vi "dfd_Classical Order Estimation Param Validation.vi"(6 "fs [Hz]":dbl=1.0 format="%.2f", 7 "filter type":T3(ring), 8 "error in (no error)":errorcluster, 10 "ripple specs":T1={"passband"=0.0, "stopband"=0.0, "dB/linear? (T: dB)"=TRUE}, 11 "freq specs [Hz]":T2) -> (0 "error out":errorcluster, 2 "dup ripple specs":T1={"passband"=0.0, "stopband"=0.0, "dB/linear? (T: dB)"=TRUE}, 3 "dup freq specs [Hz]":T2)   [LabVIEW 2017, in "NI_DigFilterLicensed.lvlib"]
doc: "Validates the parameters for order estimation."
uses:
  <vilib>/addons/Digital Filter Design/NI_DigFilterLicensed.lvlib
  <vilib>/addons/Digital Filter Design/_Objects.llb/DFD Filter Frequence Specification (Design).ctl
  <vilib>/addons/Digital Filter Design/_Objects.llb/DFD Filter Ripple Specification (Design).ctl
  <vilib>/addons/Digital Filter Design/_Misc.llb/dfd_Error Handlers (Multiple).vi
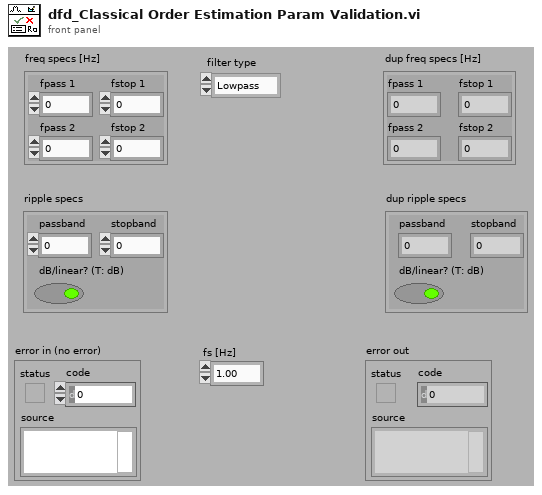
[diagram p1: front panel]
types:
  T1 = typedef "NI_DigFilterLicensed.lvlib/DFD Filter Ripple Specification (Design).ctl" = cluster{"passband":dbl, "stopband":dbl, "dB/linear? (T: dB)":bool}
  T2 = typedef "NI_DigFilterLicensed.lvlib/DFD Filter Frequence Specification (Design).ctl" = cluster{"fpass 1":dbl, "fstop 1":dbl, "fpass 2 ":dbl, "fstop 2":dbl}
  T3 = enum16{"Lowpass", "Highpass", "Bandpass", "Bandstop"}
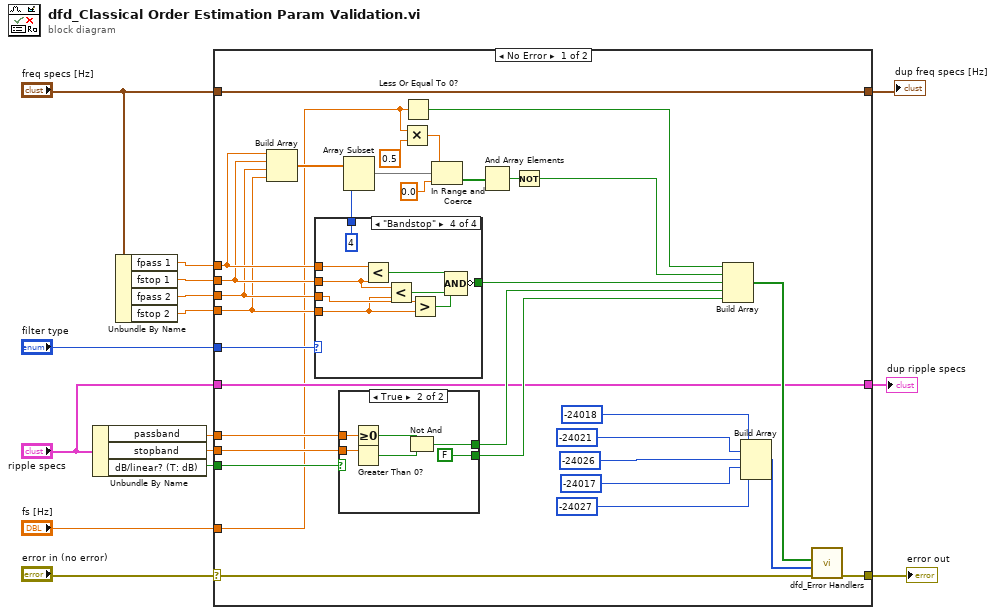
[diagram p0: block diagram]
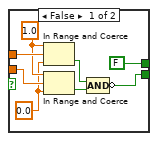
[diagram p2: hidden frame]
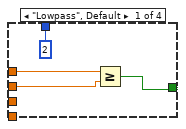
[diagram p3: hidden frame]
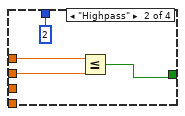
[diagram p4: hidden frame]
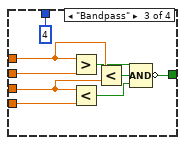
[diagram p5: hidden frame]
diagram:
  n1 = Unbundle By Name("ripple specs") -> ("passband"=w8:dbl, "stopband"=w7:dbl, "dB/linear? (T: dB)"=w9:bool)
  n2 = Unbundle By Name("freq specs [Hz]") -> ("fpass 1"=w13:dbl, "fstop 1"=w12:dbl, "fpass 2"=w11:dbl, "fstop 2"=w10:dbl)
  n3 = case shown="No Error" "error in (no error)" {
    selector: "error in (no error)" -> [w32 w89]
    tunnel: "fs [Hz]" -> [w26 _]
    tunnel: "filter type" -> [w48 _]
    tunnel: w13 -> [w42 _]
    tunnel: w12 -> [w41 _]
    tunnel: w11 -> [w40 _]
    tunnel: w10 -> [w39 _]
    tunnel: w9 -> [w45 _]
    tunnel: w8 -> [w44 _]
    tunnel: w7 -> [w43 _]
    tunnel: [w31 w89] -> w6
    tunnel: [w30 _] -> w3
    tunnel: "freq specs [Hz]" -> [w30 _]
    tunnel: "ripple specs" -> [w29 _]
    tunnel: [w29 _] -> w1
    frame No Error {
      n4 = Build Array(w42, w41, w40, w39) -> (w28:dbl[])
      n5 = case shown="\"Bandstop\"" w48 {
        tunnel: w42 -> [w66 w70 w77 w88]
        tunnel: w41 -> [w65 w69 w79 w87]
        tunnel: w40 -> [_ _ w76 w86]
        tunnel: w39 -> [_ _ w78 w80]
        tunnel: [w64 w68 w72 w82] -> w47
        tunnel: [2 2 4 4] -> w27
        frame "Lowpass", Default {
          n6 = Greater Or Equal?(x=w66, y=w65) -> (x >= y?=w64:bool)
        }
        frame "Highpass" {
          n7 = Less Or Equal?(x=w70, y=w69) -> (x <= y?=w68:bool)
        }
        frame "Bandpass" {
          n8 = Greater?(x=w77, y=w79) -> (0:w75:bool)
          n9 = Less?(x=w76, y=w78) -> (x < y?=w73:bool)
          n10 = Less?(x=w77, y=w76) -> (x < y?=w74:bool)
          n11 = Compound Arithmetic op=AND(w75, w74, w73) -> (invert w72:bool)
        }
        frame "Bandstop" {
          n12 = Less?(x=w88, y=w87) -> (x < y?=w85:bool)
          n13 = Less?(x=w87, y=w80) -> (x < y?=w84:bool)
          n14 = Greater?(x=w86, y=w80) -> (0:w83:bool)
          n15 = Compound Arithmetic op=AND(w85, w84, w83) -> (invert w82:bool)
        }
      }
      n16 = case shown="True" w45 {
        tunnel: w44 -> [w54 w62]
        tunnel: w43 -> [w55 w61]
        tunnel: [FALSE w58] -> w36
        tunnel: [w49 FALSE] -> w35
        frame False {
          w52 = 0.0 ("lower limit")
          w53 = 1.0 ("y")
          n17 = In Range and Coerce(upper limit=w53, x=w54, lower limit=w52) -> (In Range?=w51:bool)  [unwired: 1 out]
          n18 = In Range and Coerce(upper limit=w53, x=w55, lower limit=w52) -> (In Range?=w50:bool)  [unwired: 1 out]
          n19 = Compound Arithmetic op=AND(w51, w50) -> (invert w49:bool)
        }
        frame True {
          n20 = Greater Or Equal To 0?(x=w62) -> (x >= 0?=w60:bool)
          n21 = Greater Than 0?(x=w61) -> (x > 0?=w59:bool)
          n22 = Not And(1:w59, 2:w60) -> (0:w58:bool)
        }
      }
      n23 = Array Subset(array=w28, length=w27) -> (w24:dbl[])  [unwired: 1 in]
      n24 = Multiply(x=w26, y=0.5) -> (x*y=w17:dbl)
      n25 = Less Or Equal To 0?(x=w26) -> (x <= 0?=w18:bool)
      n26 = In Range and Coerce(upper limit=w17, x=w24, lower limit=0.0) -> (In Range?=w23:bool[])  [unwired: 1 out]
      n27 = And Array Elements(Boolean array=w23) -> (logical AND=w22:bool)
      n28 = Not(x=w22) -> (.not. x?=w21:bool)
      n29 = Build Array(w18, w21, w47, w36, w35) -> (w33:bool[])
      n30 = Build Array(-24018 ("ERR_FS_LE_ZERO"), -24021 ("ERR_FREQ_RANGE_WRONG"), -24026 ("ERR_FREQ_SEQ_WRONG"), -24017 ("ERR_dB_LE_ZERO"), -24027 ("ERR_RIPPLE_RANGE_WRONG")) -> (w34:i32[])
      n31 = call-poly <vilib>:"dfd_Error Handlers.vi"("error in (no error)"=w32, "error sources"=w34, "condition failed?"=w33) -> ("error out"=w31:errorcluster)  [unwired: 8 out]
    }
    frame Error {
    }
  }
  "error out" <- w6
  "dup freq specs [Hz]" <- w3
  "dup ripple specs" <- w1
